vi "UV-vis HP 8452A_V2.vi"() -> (1 "variance":ext[](array[numeric]) format="%.3e", 2 "measurement":ext[](array[numeric]) format="%.3e", 5 "Integration time":ext=0.5 format="%.1f", 6 "stop":ext=820.0, 7 "start":ext=190.0)   [LabVIEW 2010]
panel:
  in  "TIME BETWEEN MEASUREMENTS":bool
  in  "INTEGRATION TIME":bool
  in  "STOP":bool
  in  "START":bool
  in  "# OF SPECTRA":bool
  in  "MANUAL":bool
  out "# of spectra":dbl=1.0
  in  "STOP":bool
  in  "CLR ERRORS":bool
  in  "MEASURE":bool
  in  "REFERENCE":bool
  in  "INITIALIZE":bool
  out "Absorption spectrum":cluster{"Value Out":dbl, ext, ext[][]}(graph)
  out "Time between measurements":dbl
  out "Error":ext
  # "Wavelength range (nm)"
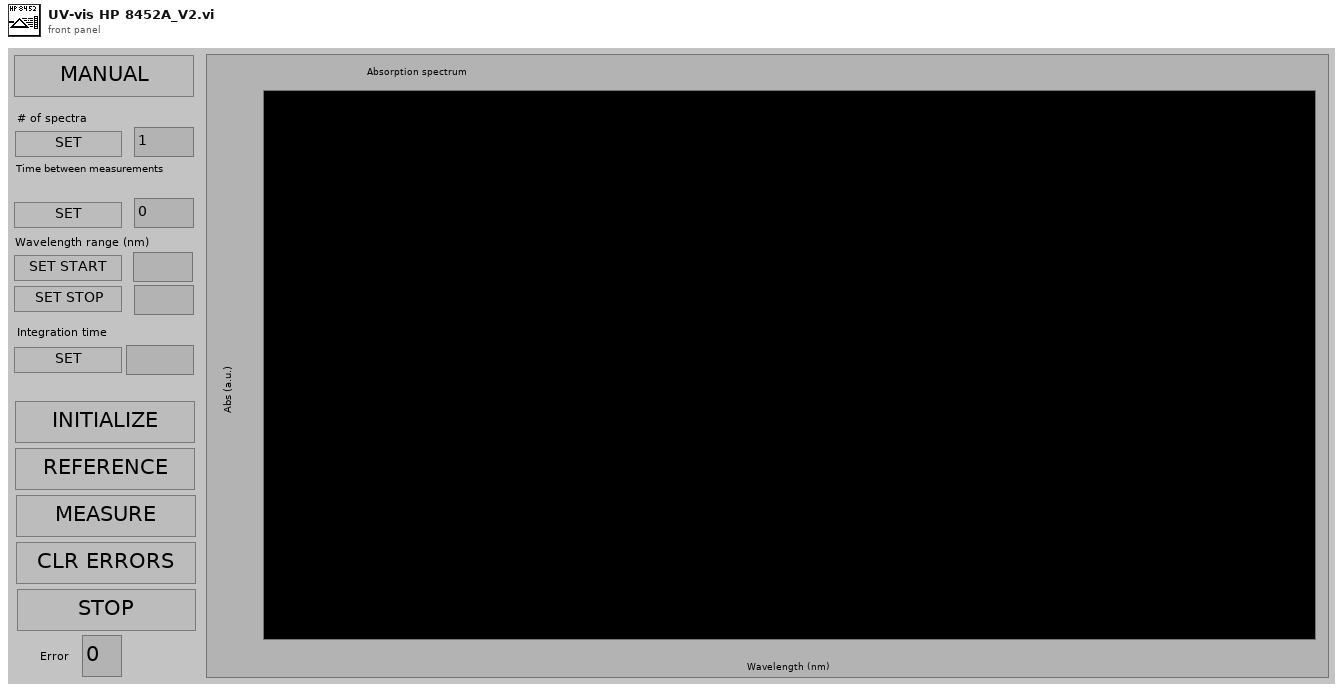
[diagram p1: front panel]
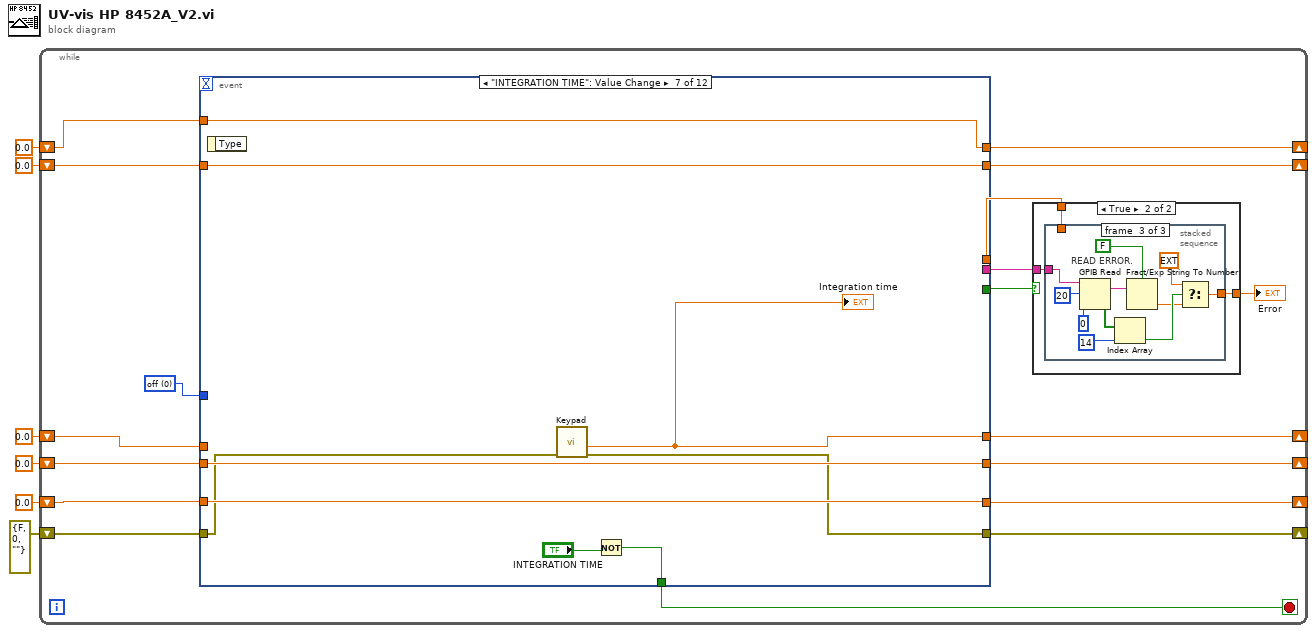
[diagram p0: block diagram]
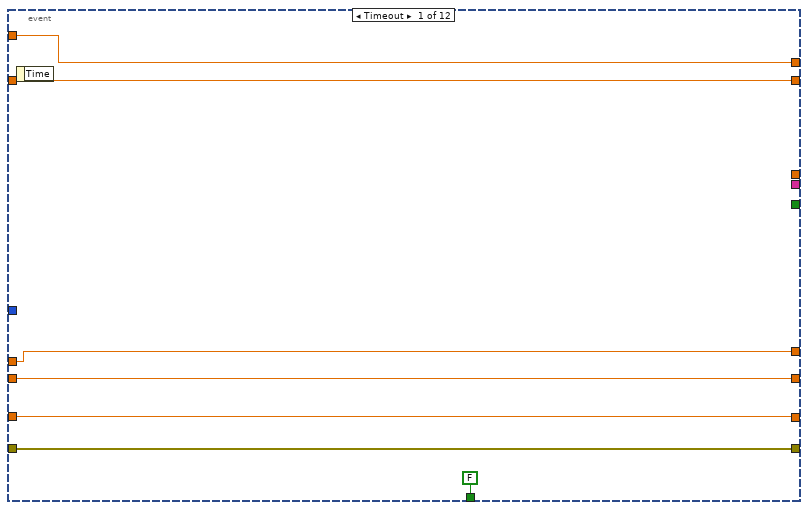
[diagram p2: hidden frame]
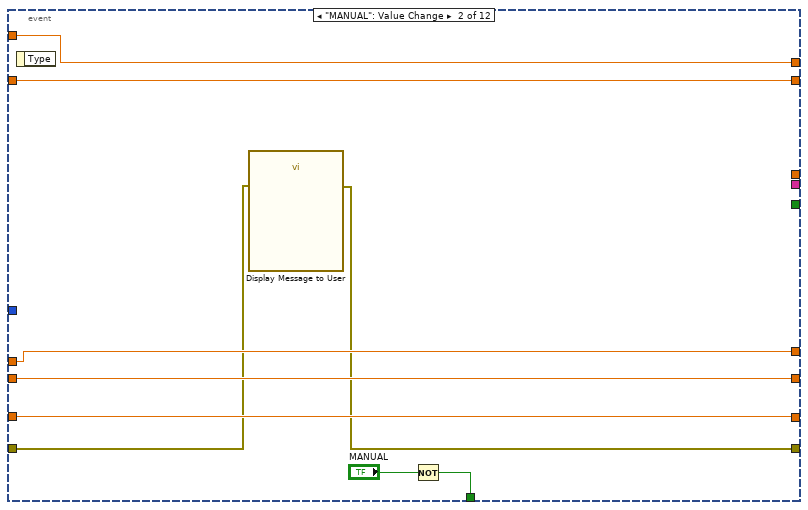
[diagram p3: hidden frame]
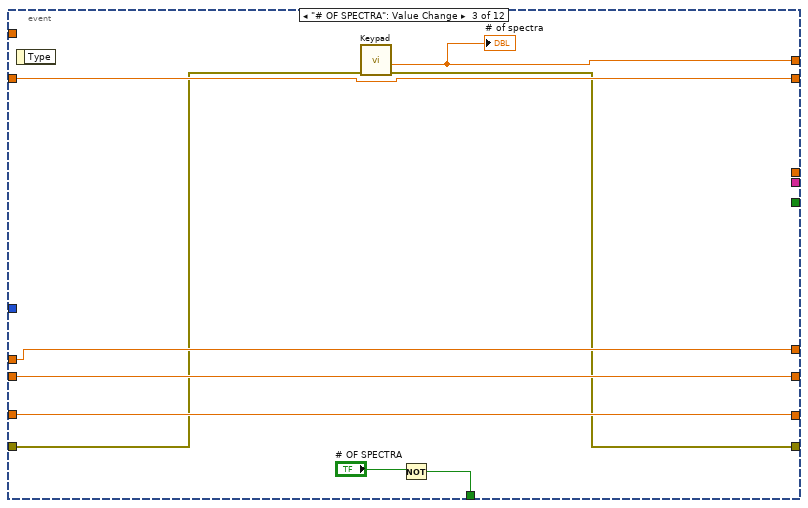
[diagram p4: hidden frame]
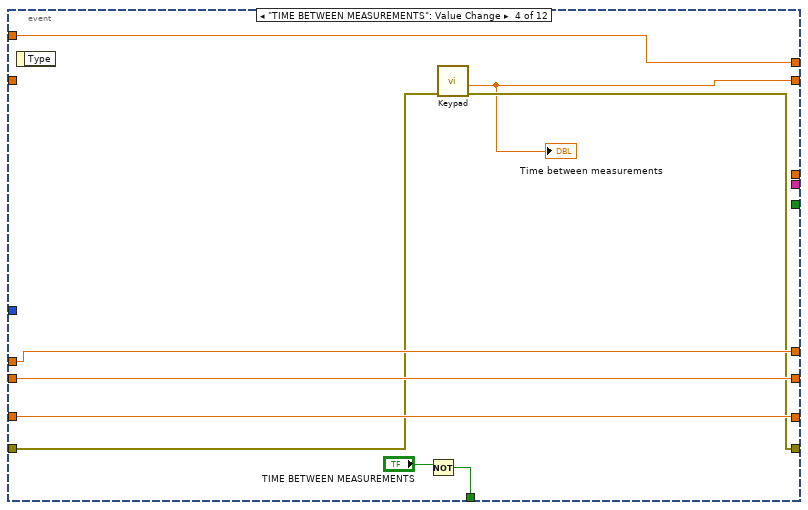
[diagram p5: hidden frame]
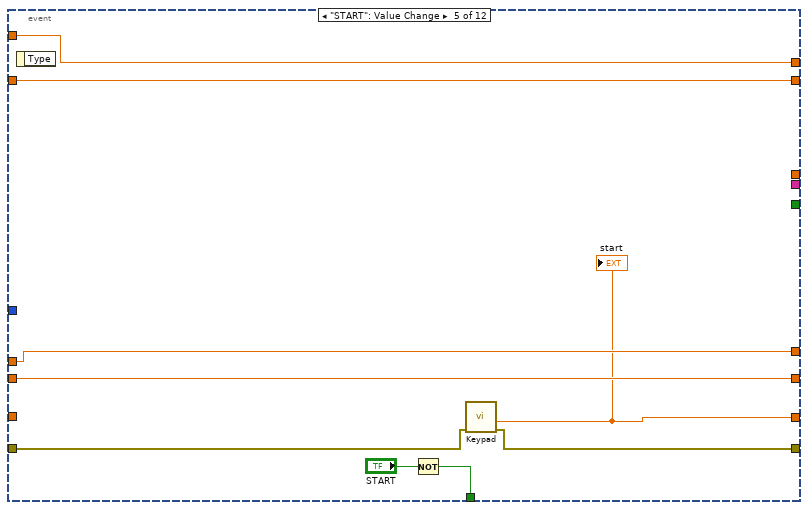
[diagram p6: hidden frame]
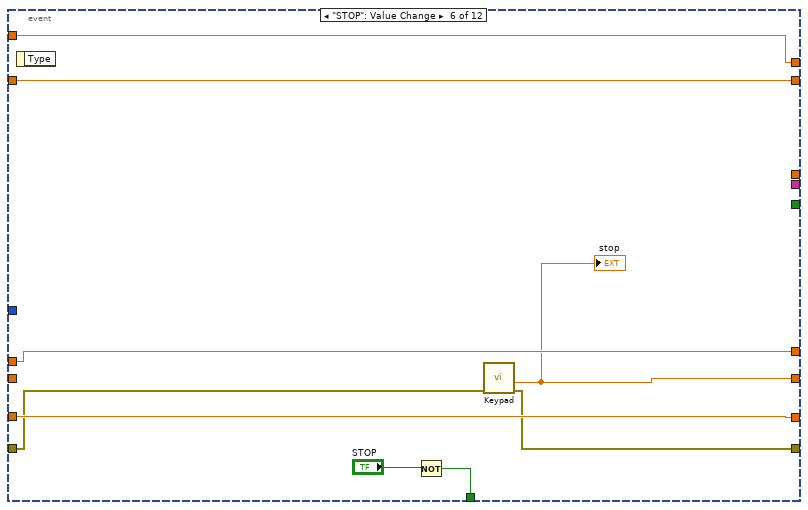
[diagram p7: hidden frame]
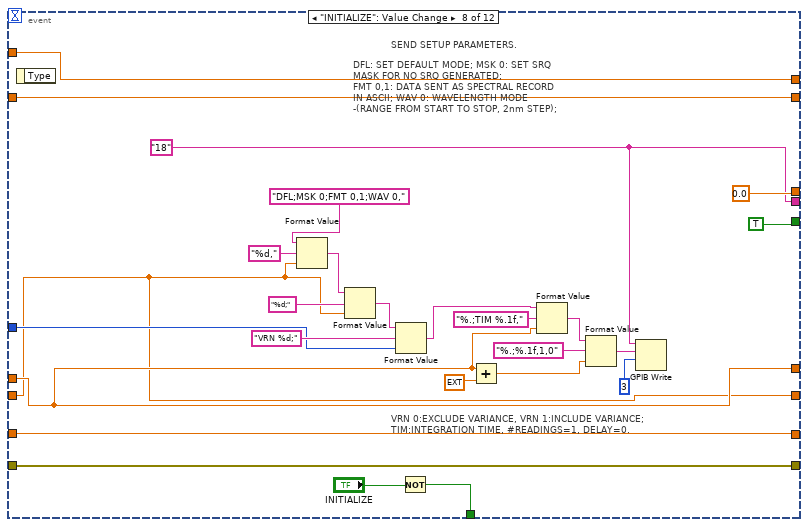
[diagram p8: hidden frame]
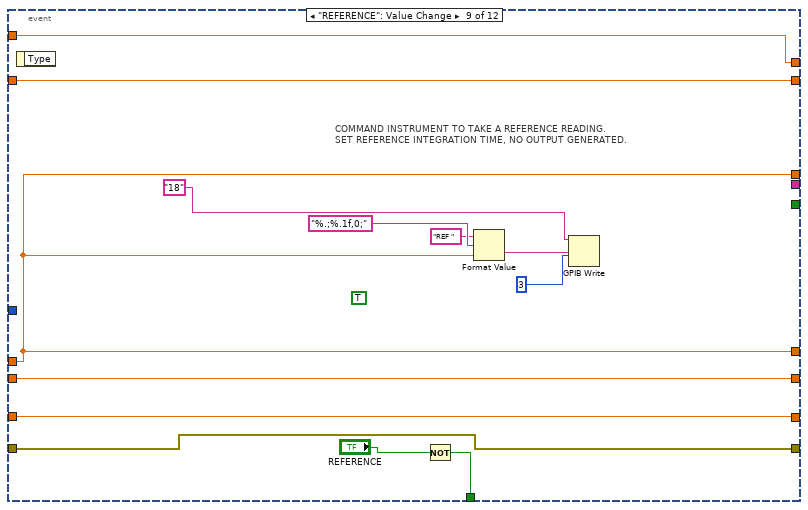
[diagram p9: hidden frame]
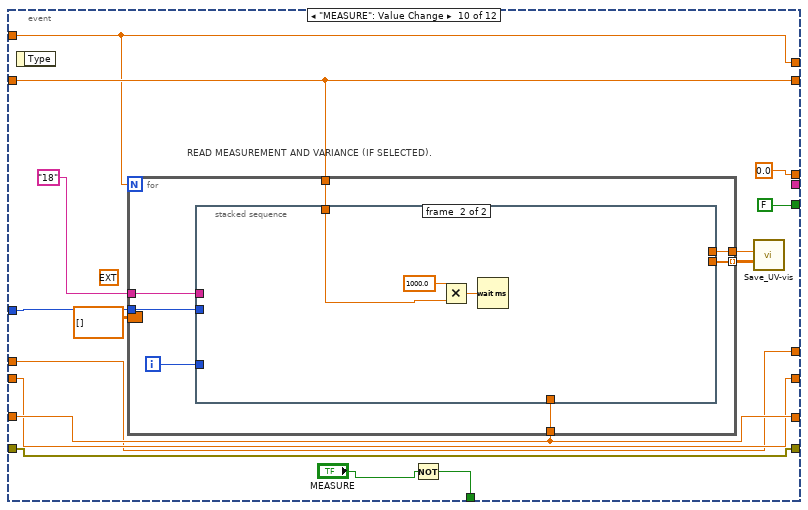
[diagram p10: hidden frame]
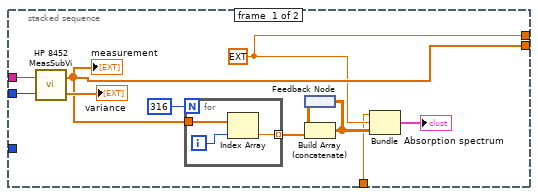
[diagram p11: hidden frame]
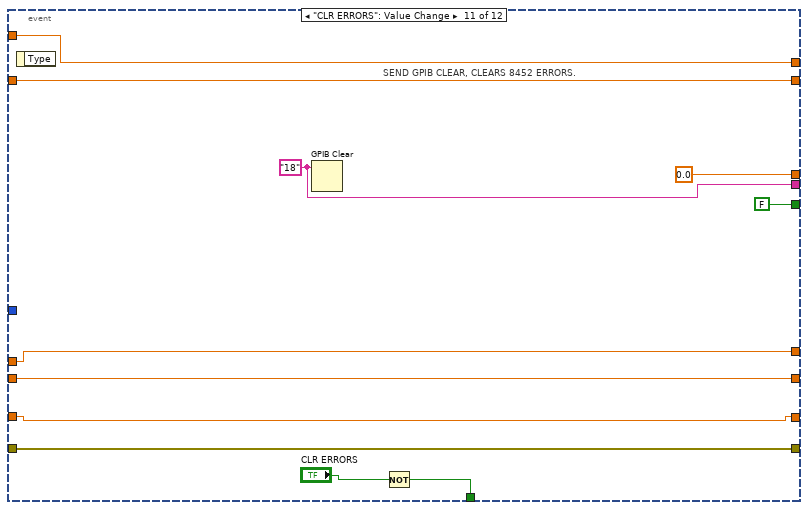
[diagram p12: hidden frame]
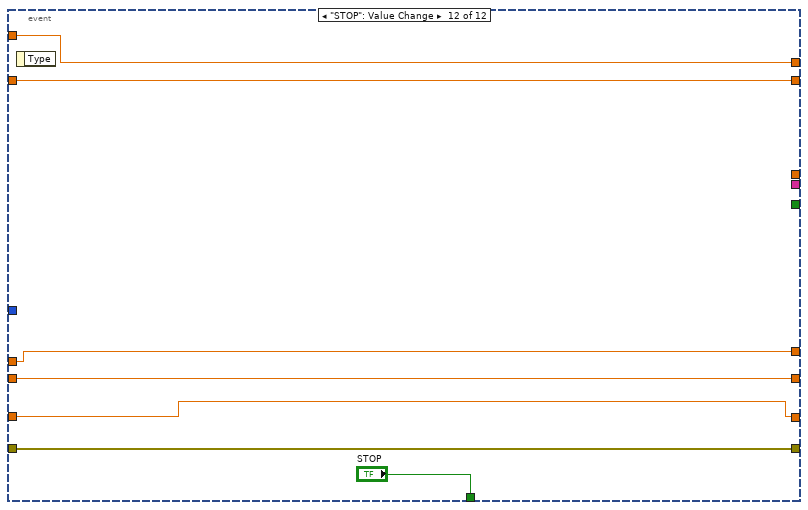
[diagram p13: hidden frame]
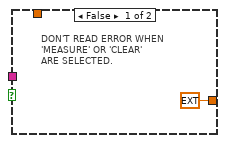
[diagram p14: hidden frame]
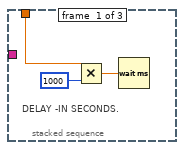
[diagram p15: hidden frame]
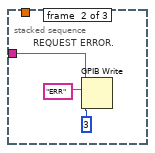
[diagram p16: hidden frame]
diagram:
  n1 = while {
    shift-right: [w18] -> _
    shift-left: 0.0 ("Value Out") -> [w16]
    shift-right: [w17] -> _
    shift-left: 0.0 ("Value Out") -> [w9]
    shift-right: [w15] -> _
    shift-left: 0.0 ("Value Out") -> [w14]
    shift-right: [w13] -> _
    shift-left: 0.0 ("Value Out") -> [w8]
    shift-right: [w12] -> _
    shift-left: 0.0 ("Value Out") -> [w7]
    shift-right: [w10] -> _
    shift-left: errorcluster {"status"=FALSE, "code"=0, "source"=""} ("error in") -> [w11]
    stop <- w19 stop-if-true
    w20 = u16 0 items=["off", "on"] ("variance (off:0)")
    n2 = event shown="[6] \"INTEGRATION TIME\": Value Change" {
      selector: _ -> [_ _ _ _ _ _ _ _ _ _ _ _]
      dyn-events: _ -> [_ _ _ _ _ _ _ _ _ _ _ _]
      timeout: _ -> [_ _ _ _ _ _ _ _ _ _ _ _]
      tunnel: [_ _ _ _ _ _ _ TRUE _ FALSE FALSE _] -> w23
      tunnel: [_ _ _ _ _ _ _ 0.0 w113 0.0 0.0 _] -> w22
      tunnel: [_ _ _ _ _ _ _ w95 _ _ w172 _] -> w21
      tunnel: w20 -> [_ _ _ _ _ _ _ w94 _ w133 _ _]
      tunnel: [FALSE ("STOP") w39 w44 w53 w63 w71 w80 w92 w118 w131 w171 "STOP"] -> w19
      tunnel: [w30 w38 w41 w58 w67 w76 w85 w91 w117 w129 w169 w180] -> w18
      tunnel: [w29 w37 w49 w50 w66 w75 w84 w90 w116 w130 w168 w179] -> w17
      tunnel: w9 -> [w29 w37 w49 _ w66 w75 w84 w90 w116 w130 w168 w179]
      tunnel: w16 -> [w30 w38 _ w58 w67 w76 w85 w91 w117 w129 w169 w180]
      tunnel: [w28 w36 w48 w57 w59 w74 w83 w89 w115 w128 w167 w178] -> w15
      tunnel: w14 -> [w28 w36 w48 w57 _ w74 w83 w89 w115 w128 w167 w178]
      tunnel: [w27 w35 w47 w56 w65 w68 w82 w86 w114 w127 w166 w177] -> w13
      tunnel: w8 -> [w27 w35 w47 w56 w65 _ w82 w86 w114 w127 w166 w177]
      tunnel: [w26 w34 w46 w55 w64 w73 w77 w88 w113 w126 w165 w176] -> w12
      tunnel: w7 -> [w26 w34 w46 w55 w64 w73 _ w88 w113 w126 w165 w176]
      tunnel: w11 -> [w25 w33 w43 w52 w61 w70 w79 w87 w112 w125 w164 w175]
      tunnel: [w25 w32 w42 w51 w60 w69 w78 w87 w112 w125 w164 w175] -> w10
      event Timeout {
        n3 = event-data() -> ()  [unwired: 1 in, 1 out]
      }
      event "MANUAL": Value Change {
        n4 = event-data() -> ()  [unwired: 1 in, 1 out]
        n5 = call "Display Message to User"("error in (no error)"=w33) -> ("error out"=w32:errorcluster)  [unwired: 9 in, 1 out]
        n6 = Not(x="MANUAL") -> (.not. x?=w39:bool)
      }
      event "# OF SPECTRA": Value Change {
        n7 = event-data() -> ()  [unwired: 1 in, 1 out]
        n8 = call <userlib>:"Keypad.vi"("error in (no error)"=w43) -> ("error out"=w42:errorcluster, "Value Out"=w41:dbl)  [unwired: 5 in]
        "# of spectra" <- w41
        n9 = Not(x="# OF SPECTRA") -> (.not. x?=w44:bool)
      }
      event "TIME BETWEEN MEASUREMENTS": Value Change {
        n10 = event-data() -> ()  [unwired: 1 in, 1 out]
        n11 = Not(x="TIME BETWEEN MEASUREMENTS") -> (.not. x?=w53:bool)
        n12 = call <userlib>:"Keypad.vi"("error in (no error)"=w52) -> ("error out"=w51:errorcluster, "Value Out"=w50:dbl)  [unwired: 5 in]
        "Time between measurements" <- w50
      }
      event "START": Value Change {
        n13 = event-data() -> ()  [unwired: 1 in, 1 out]
        n14 = Not(x="START") -> (.not. x?=w63:bool)
        n15 = call <userlib>:"Keypad.vi"("error in (no error)"=w61) -> ("error out"=w60:errorcluster, "Value Out"=w59:dbl)  [unwired: 5 in]
        "start" <- w59
      }
      event "STOP": Value Change {
        n16 = event-data() -> ()  [unwired: 1 in, 1 out]
        n17 = Not(x="STOP") -> (.not. x?=w71:bool)
        n18 = call <userlib>:"Keypad.vi"("error in (no error)"=w70) -> ("error out"=w69:errorcluster, "Value Out"=w68:dbl)  [unwired: 5 in]
        "stop" <- w68
      }
      event "INTEGRATION TIME": Value Change {
        n19 = event-data() -> ()  [unwired: 1 in, 1 out]
        n20 = call <userlib>:"Keypad.vi"("error in (no error)"=w79) -> ("error out"=w78:errorcluster, "Value Out"=w77:dbl)  [unwired: 5 in]
        "Integration time" <- w77
        n21 = Not(x="INTEGRATION TIME") -> (.not. x?=w80:bool)
      }
      event "INITIALIZE": Value Change {
        w95 = "18"
        # "VRN 0:EXCLUDE VARIANCE, VRN 1:INCLUDE VARIANCE;\nTIM:INTEGRATION TIME, #READINGS=1, DELAY=0."
        # "DFL: SET DEFAULT MODE; MSK 0: SET SRQ\nMASK FOR NO SRQ GENERATED;\nFMT 0,1: DATA SENT AS SPECTRAL RECORD\nIN ASCII; WAV 0: WAVELENGTH MODE\n-(RANGE FROM START TO STOP, 2nm STEP);"
        # "SEND SETUP PARAMETERS."
        n22 = event-data() -> ()  [unwired: 1 in, 1 out]
        n23 = Format Value(string ("")="DFL;MSK 0;FMT 0,1;WAV 0,", format string="%d,", value (0)=w86) -> (output string=w107:string)
        n24 = Format Value(string ("")=w107, format string="%d;", value (0)=w86) -> (output string=w105:string)
        n25 = Format Value(string ("")=w105, format string="VRN %d;", value (0)=w94) -> (output string=w102:string)
        n26 = Not(x="INITIALIZE") -> (.not. x?=w92:bool)
        n27 = Add(x=w88, y=ext 0.5) -> (x+y=w98:ext)
        n28 = Format Value(string ("")=w102, format string="%.;TIM %.1f,", value (0)=w88) -> (output string=w100:string)
        n29 = Format Value(string ("")=w100, format string="%.;%.1f,1,0", value (0)=w98) -> (output string=w97:string)
        n30 = GPIB Write(0:w95, 1:w97, 2:3) -> ()  [unwired: 2 in, 2 out]
      }
      event "REFERENCE": Value Change {
        (unwired) TRUE
        # "COMMAND INSTRUMENT TO TAKE A REFERENCE READING.\nSET REFERENCE INTEGRATION TIME, NO OUTPUT GENERATED."
        n31 = event-data() -> ()  [unwired: 1 in, 1 out]
        n32 = Not(x="REFERENCE") -> (.not. x?=w118:bool)
        n33 = Format Value(string ("")="REF ", format string="%.;%.1f,0;", value (0)=w113) -> (output string=w124:string)
        n34 = GPIB Write(0:"18", 1:w124, 2:3) -> ()  [unwired: 2 in, 2 out]
      }
      event "MEASURE": Value Change {
        (unwired) ext 0.0
        # "READ MEASUREMENT AND VARIANCE (IF SELECTED)."
        n35 = event-data() -> ()  [unwired: 1 in, 1 out]
        n36 = for {
          N: w129 -> [_]
          tunnel: "18" -> [w146]
          tunnel: w133 -> [w145]
          tunnel: [w144] -> w135
          tunnel: [w143] -> w136 mode=indexing
          border: ext[][] [] -> [_]
          tunnel: w130 -> [w141]
          tunnel: w128 -> [w140]
          i -> [w142]
          n37 = stacked-sequence {
            tunnel: w146 -> [w157 _]
            tunnel: w145 -> [w155 _]
            tunnel: [w150 _] -> w144
            tunnel: [w153 _] -> w143
            tunnel: w142 -> [_ _]
            tunnel: w141 -> [_ w161]
            tunnel: w140 -> [w147 _]
            frame #0 {
              w150 = ext 2.0
              n38 = call <instrlib>:"HP 8452 MeasSubVi.vi"("variance option (off:0)"=w155, "GPIB"=w157) -> ("variance"=→"variance":ext[], "measurement"=w153:ext[])
              "measurement" <- w153
              n39 = for {
                N: 316 -> [_]
                tunnel: w153 -> [w160]
                tunnel: [w158] -> w152 mode=indexing
                i -> [w159]
                n40 = Index Array(array=w160, index=w159) -> (element=w158:ext)
              }
              n41 = feedback #1() -> (w151:ext[][])
              n42 = Build Array (concatenate)(w151, w152) -> (w149:ext[][])
              n43 = feedback-in #1(w149) -> ()
              n44 = Bundle("Value Out"=w147, w150, w149) -> (→"Absorption spectrum":cluster{"Value Out":dbl, ext, ext[][]})  [unwired: 1 in]
            }
            frame #1 {
              n45 = Multiply(x=1000.0, y=w161) -> (x*y=w162:dbl)
              n46 = Wait (ms)(milliseconds to wait=w162) -> ()  [unwired: 1 out]
            }
          }
        }
        n47 = Not(x="MEASURE") -> (.not. x?=w131:bool)
        n48 = call <instrlib>:"Save_UV-vis.vi"("measurement"=w136, "step"=w135) -> ()  [unwired: 9 in, 1 out]
      }
      event "CLR ERRORS": Value Change {
        w172 = "18"
        # "SEND GPIB CLEAR, CLEARS 8452 ERRORS."
        n49 = event-data() -> ()  [unwired: 1 in, 1 out]
        n50 = GPIB Clear(3:w172) -> ()  [unwired: 1 in, 2 out]
        n51 = Not(x="CLR ERRORS") -> (.not. x?=w171:bool)
      }
      event "STOP": Value Change {
        n52 = event-data() -> ()  [unwired: 1 in, 1 out]
      }
    }
    n53 = case shown="True" w23 {
      tunnel: w22 -> [_ w183]
      tunnel: [ext 0.0 w184] -> w24
      tunnel: w21 -> [_ w185]
      frame False {
        # "DON'T READ ERROR WHEN\n'MEASURE' OR 'CLEAR'\nARE SELECTED."
      }
      frame True {
        n54 = stacked-sequence {
          tunnel: w183 -> [w186 _ _]
          tunnel: [_ _ w201] -> w184
          tunnel: w185 -> [_ w189 w202]
          frame #0 {
            # "DELAY -IN SECONDS."
            n55 = Multiply(x=w186, y=1000) -> (x*y=w188:dbl)
            n56 = Wait (ms)(milliseconds to wait=w188) -> ()  [unwired: 1 out]
          }
          frame #1 {
            # "REQUEST ERROR."
            n57 = GPIB Write(0:w189, 1:"ERR", 2:3) -> ()  [unwired: 2 in, 2 out]
          }
          frame #2 {
            # "READ ERROR."
            n58 = GPIB Read(0:w202, 1:20, 2:0) -> (5:w195:string, 6:w196:bool[])  [unwired: 2 in, 1 out]
            n59 = Index Array(array=w196, index=14) -> (element=w199:bool)
            n60 = Fract/Exp String To Number(use system decimal point (T)=FALSE, string=w195) -> (number=w198:dbl)  [unwired: 2 in, 1 out]
            n61 = Select(t=ext -1.0, s=w199, f=w198) -> (s? t:f=w201:ext)
          }
        }
      }
    }
    "Error" <- w24
  }
